vi "SSC DCPower Set Current.vi"(0 "DCPower SSC in":T1[](array[typedef]), 11 "error in":errorcluster, 12 "Current Level Range (A)":dbl=0.001 format="%#_13p", 14 "Current Level (A)":dbl format="%#_13g") -> (4 "DCPower SSC out":T1[](array[typedef]), 15 "error out":errorcluster)   [LabVIEW 2019]
uses:
  Instrument Control/DCPower/SSC DCPower/SSC DCPower.ctl
  <instrlib>/niDCPower/nidcpower.llb/niDCPower Output Function.ctl
  <instrlib>/niDCPower/nidcpower.llb/niDCPower Source Mode.ctl
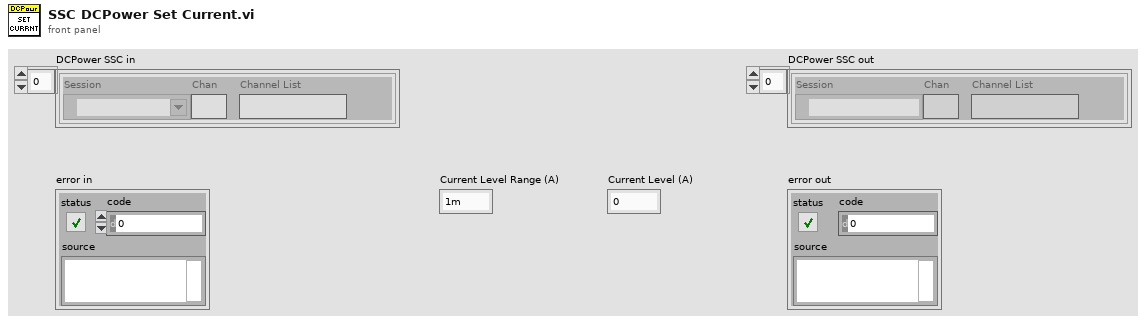
[diagram p1: front panel]
types:
  T1 = typedef "SSC DCPower.ctl" = cluster{"Session":refnum<k15>, "Chan":string, "Channel List":string}
  T2 = typedef "niDCPower Source Mode.ctl" = i32
  T3 = typedef "niDCPower Output Function.ctl" = i32
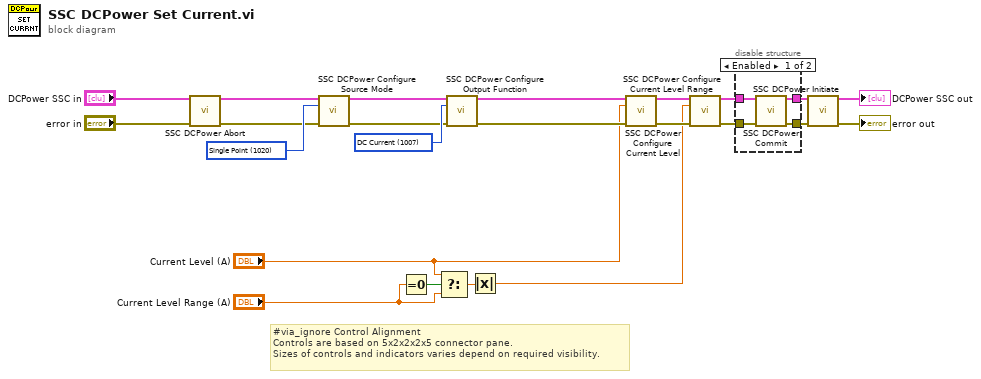
[diagram p0: block diagram]
diagram:
  w5 = T2 1020 items=["Single Point"=1020, "Sequence"=1021] ("Source Mode")
  w23 = T3 1007 items=["DC Voltage"=1006, "DC Current"=1007, "Pulse Voltage"=1049, "Pulse Current"=1050] ("Output Function")
  # "#via_ignore Control Alignment\nControls are based on 5x2x2x2x5 connector pane.\nSizes of controls and indicators varies depend on required visibility."
  n1 = call "SSC DCPower Abort.vi"("DCPower SSC in"="DCPower SSC in", "error in"="error in") -> ("DCPower SSC out"=w2:T1[], "error out"=w4:errorcluster)  [unwired: 12 in]
  n2 = call "SSC DCPower Configure Source Mode.vi"("DCPower SSC in"=w2, "Source Mode"=w5, "error in"=w4) -> ("DCPower SSC out"=w1:T1[], "error out"=w3:errorcluster)  [unwired: 11 in]
  n3 = Equal To 0?(x="Current Level Range (A)") -> (x = 0?=w10:bool)
  n4 = Select(t="Current Level (A)", s=w10, f="Current Level Range (A)") -> (s? t:f=w7:dbl)
  n5 = call "SSC DCPower Configure Output Function.vi"("DCPower SSC in"=w1, "Output Function"=w23, "error in"=w3) -> ("DCPower SSC out"=w21:T1[], "error out"=w20:errorcluster)  [unwired: 11 in]
  n6 = Absolute Value(x=w7) -> (abs(x)=w6:dbl)
  n7 = call "SSC DCPower Configure Current Level.vi"("DCPower SSC in"=w21, "Current Level (A)"="Current Level (A)", "error in"=w20) -> ("DCPower SSC out"=w19:T1[], "error out"=w18:errorcluster)  [unwired: 11 in]
  n8 = call "SSC DCPower Configure Current Level Range.vi"("DCPower SSC in"=w19, "Current Level Range (A)"=w6, "error in"=w18) -> ("DCPower SSC out"=w14:T1[], "error out"=w17:errorcluster)  [unwired: 11 in]
  n9 = disable-structure shown="Enabled" {
    disable-tunnel: w17 -> [w27 w29]
    disable-tunnel: [w26 w29] -> w15
    disable-tunnel: w14 -> [w25 w28]
    disable-tunnel: [w24 w28] -> w12
    frame Enabled {
      n10 = call "SSC DCPower Commit.vi"("DCPower SSC in"=w25, "error in"=w27) -> ("DCPower SSC out"=w24:T1[], "error out"=w26:errorcluster)  [unwired: 12 in]
    }
    frame Disabled {
    }
  }
  n11 = call "SSC DCPower Initiate.vi"("DCPower SSC in"=w12, "error in"=w15) -> ("DCPower SSC out"=→"DCPower SSC out":T1[], "error out"=→"error out":errorcluster)  [unwired: 12 in]
